vi "read_pbot_vector.vi"(8 "error constant":errorcluster, 9 "disconnectPBot_Event":refnum<user-event>, 10 "settingName":string, 11 "VISA resource name":refnum<visa-resource-name>) -> (0 "error out":errorcluster, 3 "vectorOut":cluster{"X":dbl, "Y":dbl, "Z":dbl})   [LabVIEW 2015]
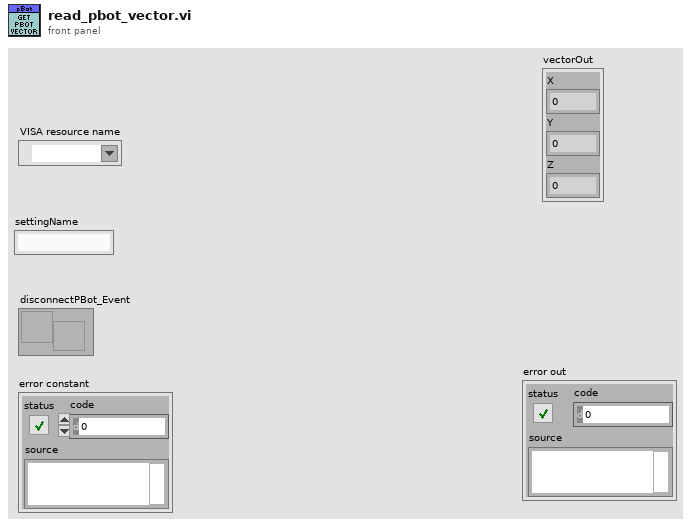
[diagram p1: front panel]
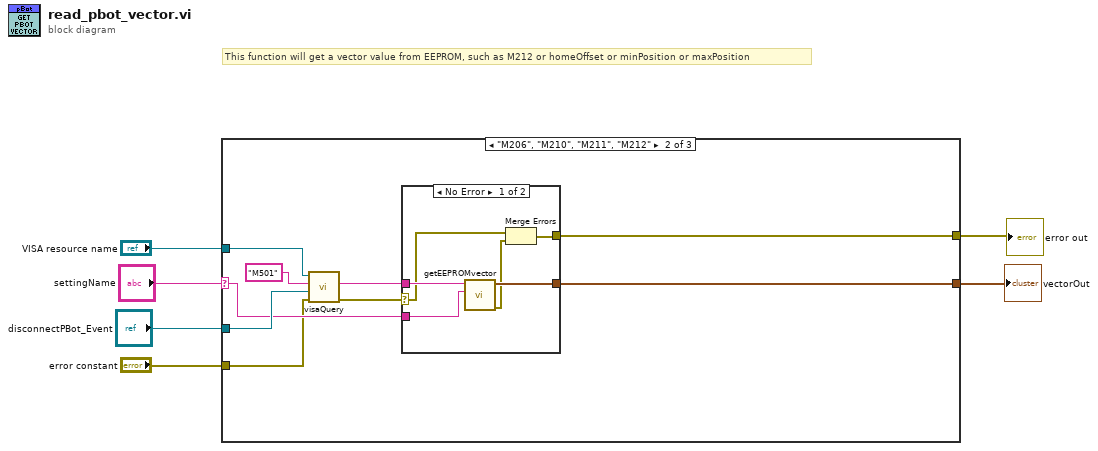
[diagram p0: block diagram]
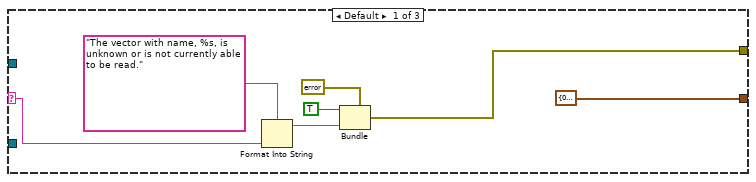
[diagram p2: hidden frame]
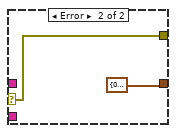
[diagram p3: hidden frame]
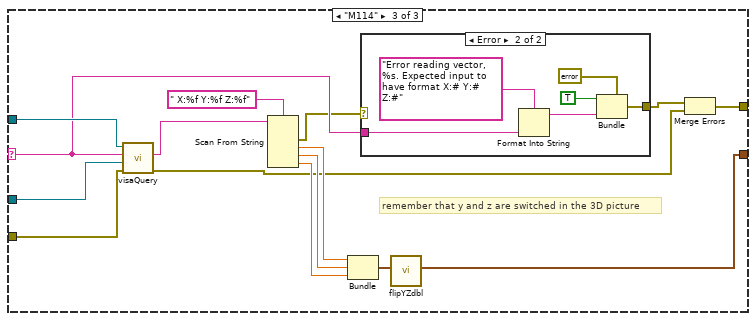
[diagram p4: hidden frame]
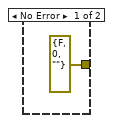
[diagram p5: hidden frame]
diagram:
  # "This function will get a vector value from EEPROM, such as M212 or homeOffset or minPosition or maxPosition"
  n1 = case shown="\"M206\", \"M210\", \"M211\", \"M212\"" "settingName" {
    selector: "settingName" -> [w8 w19 w37]
    tunnel: "VISA resource name" -> [_ w22 w45]
    tunnel: "disconnectPBot_Event" -> [_ w21 w44]
    tunnel: [cluster{"X":dbl, "Y":dbl, "Z":dbl} {"X"=0.0, "Y"=0.0, "Z"=0.0} ("vector") w18 w35] -> w3
    tunnel: [w7 w16 w32] -> w1
    tunnel: "error constant" -> [_ w15 w34]
    frame Default {
      n2 = Format Into String(format string="The vector with name, %s, is unknown or is not currently able to be read.", w8) -> (resulting string=w11:string)  [unwired: 2 in, 1 out]
      n3 = Bundle(cluster=errorcluster {"status"=TRUE, "code"=0, "source"=""} ("error constant"), "status"=TRUE, "source"=w11) -> (w7:errorcluster)  [unwired: 1 in]
    }
    frame "M206", "M210", "M211", "M212" {
      n4 = call "visaQuery.vi"("error constant"=w15, "disconnectPBot_Event"=w21, "stringToWrite"="M501", "VISA resource name"=w22) -> ("error Out"=w17:errorcluster, "String"=w20:string)  [unwired: 5 in, 1 out]
      n5 = case shown="No Error" w17 {
        selector: w17 -> [w24 w30]
        tunnel: w20 -> [w28 _]
        tunnel: w19 -> [w27 _]
        tunnel: [w26 cluster{"X":dbl, "Y":dbl, "Z":dbl} {"X"=0.0, "Y"=0.0, "Z"=0.0} ("vector")] -> w18
        tunnel: [w25 w30] -> w16
        frame No Error {
          n6 = call "getEEPROMvector.vi"("vectorName"=w27, "EEPROM_Settings"=w28) -> ("error out"=w23:errorcluster, "vectorOut"=w26:cluster{dbl, dbl, dbl})  [unwired: 8 in]
          n7 = Merge Errors(w24, w23) -> (w25:errorcluster)
        }
        frame Error {
        }
      }
    }
    frame "M114" {
      # "remember that y and z are switched in the 3D picture"
      n8 = call "visaQuery.vi"("error constant"=w34, "disconnectPBot_Event"=w44, "stringToWrite"=w37, "VISA resource name"=w45) -> ("error Out"=w31:errorcluster, "String"=w38:string)  [unwired: 5 in, 1 out]
      n9 = Scan From String(format string=" X:%f Y:%f Z:%f", input string=w38) -> (error out=w36:errorcluster, output 1=w40:dbl, output 2=w41:dbl, output 3=w42:dbl)  [unwired: 5 in, 2 out]
      n10 = Bundle(w40, w41, w42) -> (w43:cluster{dbl, dbl, dbl})  [unwired: 1 in]
      n11 = case shown="Error" w36 {
        tunnel: [errorcluster {"status"=FALSE, "code"=0, "source"=""} ("error constant") w47] -> w33
        tunnel: w37 -> [_ w51]
        frame No Error {
        }
        frame Error {
          n12 = Format Into String(format string="Error reading vector, %s. Expected input to have format X:# Y:# Z:#", w51) -> (resulting string=w49:string)  [unwired: 2 in, 1 out]
          n13 = Bundle(cluster=errorcluster {"status"=TRUE, "code"=0, "source"=""} ("error constant"), "status"=TRUE, "source"=w49) -> (w47:errorcluster)  [unwired: 1 in]
        }
      }
      n14 = call "flipYZdbl.vi"("pointIn"=w43) -> ("pointOut"=w35:cluster{"X":dbl, "Y":dbl, "Z":dbl})  [unwired: 10 in]
      n15 = Merge Errors(w33, w31) -> (w32:errorcluster)
    }
  }
  "error out" <- w1
  "vectorOut" <- w3
